vi "Get ID.vi"(8 "error in (no error)":errorcluster, 11 "Element Base in":refnum<class "Element Base.lvclass">) -> (0 "error out":errorcluster, 2 "ID":i32, 3 "Element Base out":refnum<class "Element Base.lvclass">)   [LabVIEW 2020, in "Array Example.lvlib" / "Element Base.lvclass"]
uses:
  Element Base.lvclass
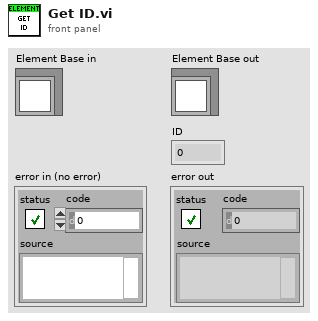
[diagram p1: front panel]
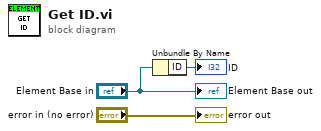
[diagram p0: block diagram]
diagram:
  n1 = Unbundle By Name("Element Base in") -> ("ID"=→"ID":i32)
  "error out" <- "error in (no error)"
  "Element Base out" <- "Element Base in"
